vi "VisualizeCHROMA1.vi"() -> ()   [LabVIEW 2018, in "Visualization.lvlib" / "VisualizeAcPwr.lvclass"]
uses:
  VisualizeAcPwr.lvclass
  VisualizeBase/VisualizeBase_class/Requests/clUserEventType.ctl
  <vilib>/event_ctls.llb/usereventprio.ctl
  <vilib>/Utility/error.llb/Error Cluster From Error Code.vi
  <vilib>/ErrorRing/Error Ring.xnode
  VisualizeBase/VisualizeBase_class/VisualizeBase.lvclass
  <userlib>/NIST/NISTErrorLib/NISTErrorLib.lvlib
  AcPwr/AcPwrModule/AcPwrModule.lvlib
panel:
  in  "Tab Control":enum32{"Chart", "XY Graph"}(tab)
  out "Chroma":waveform(dbl)[](graph)=[{"t0"=timestamp(3659455182.3010225 s since 1904-01-01), "dt"=1.0, "Y"=[17.84]}, {"t0"=timestamp(3659455182.3010225 s since 1904-01-01), "dt"=1.0, "Y"=[3.99]}]
  in  "PlotYAxis":u32[](array[numeric])=[0, 1, 0] max=1
  out "Incorrect DataType?":bool
  out "Chroma's Internal Errors/Warnings":string="No Error"
  out "XY Graph":cluster{dbl[], dbl[]}(graph)={[0.02, 0.02, 0.02, 0.02, 0.02, 0.02, 0.02, 0.02, 0.1, 0.1, 0.1, 0.1, 0.1, 0.11, 0.2, 0.2, 0.2, 0.2, 0.2, 0.2, 0.3, 0.3, 0.3, 0.3, 0.3, 0.3, 0.3, 0.37, 0.4, 0.4, 0.4, 0.4, 0.4, 0.4, 0.48, 0.5, 0.5, 0.5, 0.5, 0.5, 0.5, 0.59, 0.6, 0.6, 0.6, 0.6, 0.6, 0.6, 0.6, 0.69, 0.69, 0.69, 0.69, 0.69, 0.69, 0.71, 0.79, 0.79, 0.79, 0.79, 0.79, 0.79, 0.89, 0.89, 0.89, 0.89, 0.89, 0.89, 0.89, 1.0, 1.0, 1.0, 1.0, 1.0, 1.0, 1.0, 1.1, 1.1, 1.1, 1.09, 1.09, 1.09, 1.1, 1.19, 1.19, 1.2, 1.2, 1.2, 1.2, 1.2, 1.29, 1.29, 1.29, 1.29, 1.29, 1.29, 1.29, 1.39, 1.39, 1.39, 1.39, 1.39, 1.39, 1.39, 1.4, 1.49, 1.49, 1.49, 1.49, 1.49, 1.49, 1.57, 1.59, 1.59, 1.59, 1.59, 1.59, 1.59, 1.69, 1.69, 1.69, 1.69, 1.69, 1.69, 1.69, 1.79, 1.79, 1.79, 1.79, 1.79, 1.79, 1.79, 1.89, 1.89, 1.89, 1.89, 1.89, 1.89, 1.89, 1.99, 1.99, 1.99, 1.99, 1.99, 1.99, 2.0, 2.09, 2.09, 2.09, 2.09, 2.09, 2.09, 2.13, 2.19, 2.19, 2.19, 2.19, 2.19, 2.19, 2.29, 2.29, 2.29, 2.29, 2.29, 2.29, 2.29, 2.29, 2.39, 2.39, 2.39, 2.39, 2.39, 2.39, 2.39, 2.49, 2.49, 2.49, 2.49, 2.49, 2.49, 2.51, 2.59, 2.59, 2.59, 2.59, 2.59, 2.59, 2.69, 2.69, 2.69, 2.69, 2.69, 2.69, 2.69, 2.79, 2.79, 2.79, 2.79, 2.79, 2.79, 2.79, 2.81, 2.89, 2.89, 2.89, 2.89, 2.89, 2.89, 2.89, 2.99, 2.99, 2.99, 2.99, 2.99, 2.99, 3.0, 3.09, 3.09, 3.09, 3.09, 3.09, 3.09, 3.1, 3.19, 3.19, 3.19, 3.19, 3.19, 3.19, 3.29, 3.29, 3.29, 3.29, 3.29, 3.29, 3.29, 3.39, 3.39, 3.39, 3.39, 3.39, 3.39, 3.39, 3.39, 3.49, 3.49, 3.49, 3.49, 3.49, 3.49, 3.49, 3.5, 3.59, 3.59, 3.59, 3.59, 3.59, 3.59, 3.6, 3.69, 3.69, 3.69, 3.69, 3.69, 3.69, 3.79, 3.79, 3.79, 3.79, 3.79, 3.79, 3.79, 3.89, 3.89, 3.89, 3.89, 3.89, 3.89, 3.89, 3.99, 3.99, 3.99, 3.99, 3.99, 3.99, 3.99], [42.02, 41.83, 42.15, 41.98, 41.52, 41.47, 41.64, 41.55, 41.51, 41.49, 41.46, 41.51, 41.41, 41.39, 41.42, 41.42, 41.41, 41.4, 41.29, 41.3, 41.32, 41.33, 41.32, 41.31, 41.32, 41.21, 41.21, 41.2, 41.2, 41.21, 41.22, 41.21, 41.1, 41.1, 41.09, 41.1, 41.09, 41.11, 41.1, 40.98, 40.99, 40.98, 40.98, 40.99, 40.99, 40.98, 40.98, 40.86, 40.86, 40.88, 40.87, 40.88, 40.87, 40.87, 40.74, 40.75, 40.75, 40.75, 40.73, 40.76, 40.63, 40.63, 40.62, 40.64, 40.64, 40.61, 40.64, 40.6, 40.5, 40.46, 40.5, 40.51, 40.5, 40.51, 40.37, 40.37, 40.37, 40.37, 40.37, 40.38, 40.37, 40.36, 40.22, 40.23, 40.23, 40.24, 40.23, 40.24, 40.1, 40.09, 40.07, 40.11, 40.09, 40.09, 40.11, 39.96, 39.96, 39.95, 39.96, 39.96, 39.96, 39.94, 39.81, 39.79, 39.79, 39.81, 39.8, 39.79, 39.79, 39.81, 39.65, 39.65, 39.65, 39.65, 39.64, 39.64, 39.65, 39.48, 39.48, 39.48, 39.48, 39.47, 39.48, 39.31, 39.31, 39.3, 39.31, 39.32, 39.31, 39.31, 39.14, 39.13, 39.13, 39.14, 39.13, 39.14, 39.13, 38.95, 38.95, 38.95, 38.94, 38.95, 38.95, 38.95, 38.75, 38.75, 38.76, 38.76, 38.75, 38.75, 38.75, 38.56, 38.56, 38.56, 38.56, 38.56, 38.55, 38.34, 38.34, 38.34, 38.33, 38.33, 38.34, 38.34, 38.11, 38.11, 38.1, 38.11, 38.12, 38.1, 38.11, 38.11, 37.87, 37.86, 37.86, 37.88, 37.86, 37.88, 37.86, 37.6, 37.61, 37.61, 37.61, 37.61, 37.61, 37.62, 37.33, 37.34, 37.33, 37.34, 37.34, 37.34, 37.04, 37.04, 37.05, 37.04, 37.06, 37.05, 37.04, 36.72, 36.72, 36.71, 36.72, 36.73, 36.72, 36.71, 36.72, 36.38, 36.37, 36.39, 36.37, 36.37, 36.38, 36.37, 36.0, 36.0, 35.99, 36.0, 35.99, 36.0, 35.99, 35.59, 35.59, 35.58, 35.58, 35.58, 35.58, 35.12, 35.12, 35.12, 35.13, 35.13, 35.13, 35.12, 34.6, 34.59, 34.59, 34.59, 34.59, 34.59, 34.59, 34.6, 33.97, 33.97, 33.98, 33.97, 33.98, 33.98, 33.98, 33.26, 33.27, 33.26, 33.26, 33.26, 33.26, 33.26, 33.26, 32.38, 32.39, 32.39, 32.37, 32.37, 32.39, 32.38, 31.25, 31.24, 31.25, 31.25, 31.25, 31.25, 29.64, 29.66, 29.66, 29.67, 29.65, 29.66, 29.66, 27.14, 27.15, 27.15, 27.15, 27.14, 27.14, 27.15, 17.86, 17.84]}
  in  "PluginName":string="AcPwr.Chroma1"
  out "ErrorArray":errorcluster[](array[cluster])
  in  "QueuName":string="CHROMADCVQ"
  in  "btnStop":bool
  in  "btnReset":bool
  in  "btnClear":bool
  # "0=Left Axis and 1=Right Axis"
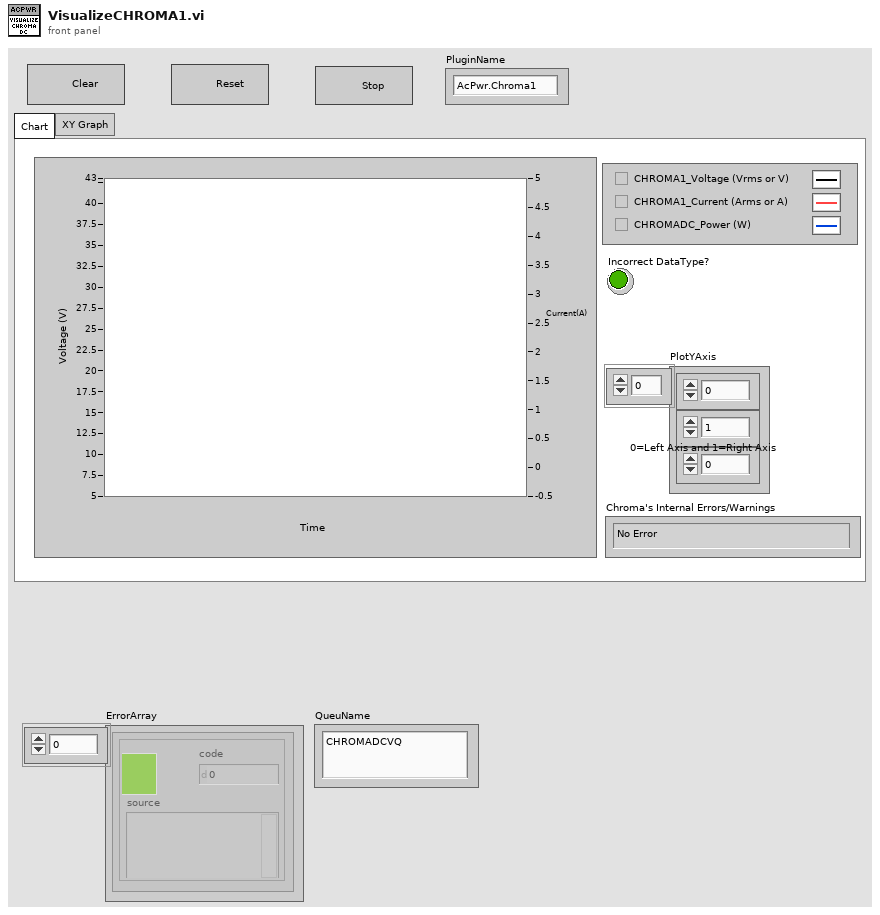
[diagram p1: front panel]
types:
  T1 = typedef "Visualization.lvlib/VisualizeBase.lvclass/clRequestEvents.ctl" = cluster{"StopRequest":refnum<user-event>, "ResetRequest":refnum<user-event>}
  T2 = typedef "AcPwrModule.lvlib/clBroadcastEvents.ctl" = cluster{"DidInit":refnum<user-event>, "StatusUpdate":refnum<user-event>, "ErrorReport":refnum<user-event>, "DidStop":refnum<user-event>, "PathToINI":refnum<user-event>, "Measurements":refnum<user-event>, "LoadConfigFile":refnum<user-event>, "GetSettings":refnum<user-event>, "SetSettings":refnum<user-event>, "GetType&ID":refnum<user-event>, "GotSettings":refnum<user-event>}
  T3 = typedef "Visualization.lvlib/VisualizeBase.lvclass/clUserEventType.ctl" = cluster{"BusIndex":i8, "Data":variant}
  T4 = typedef "usereventprio.ctl" = enum32{"high priority", "normal priority"}
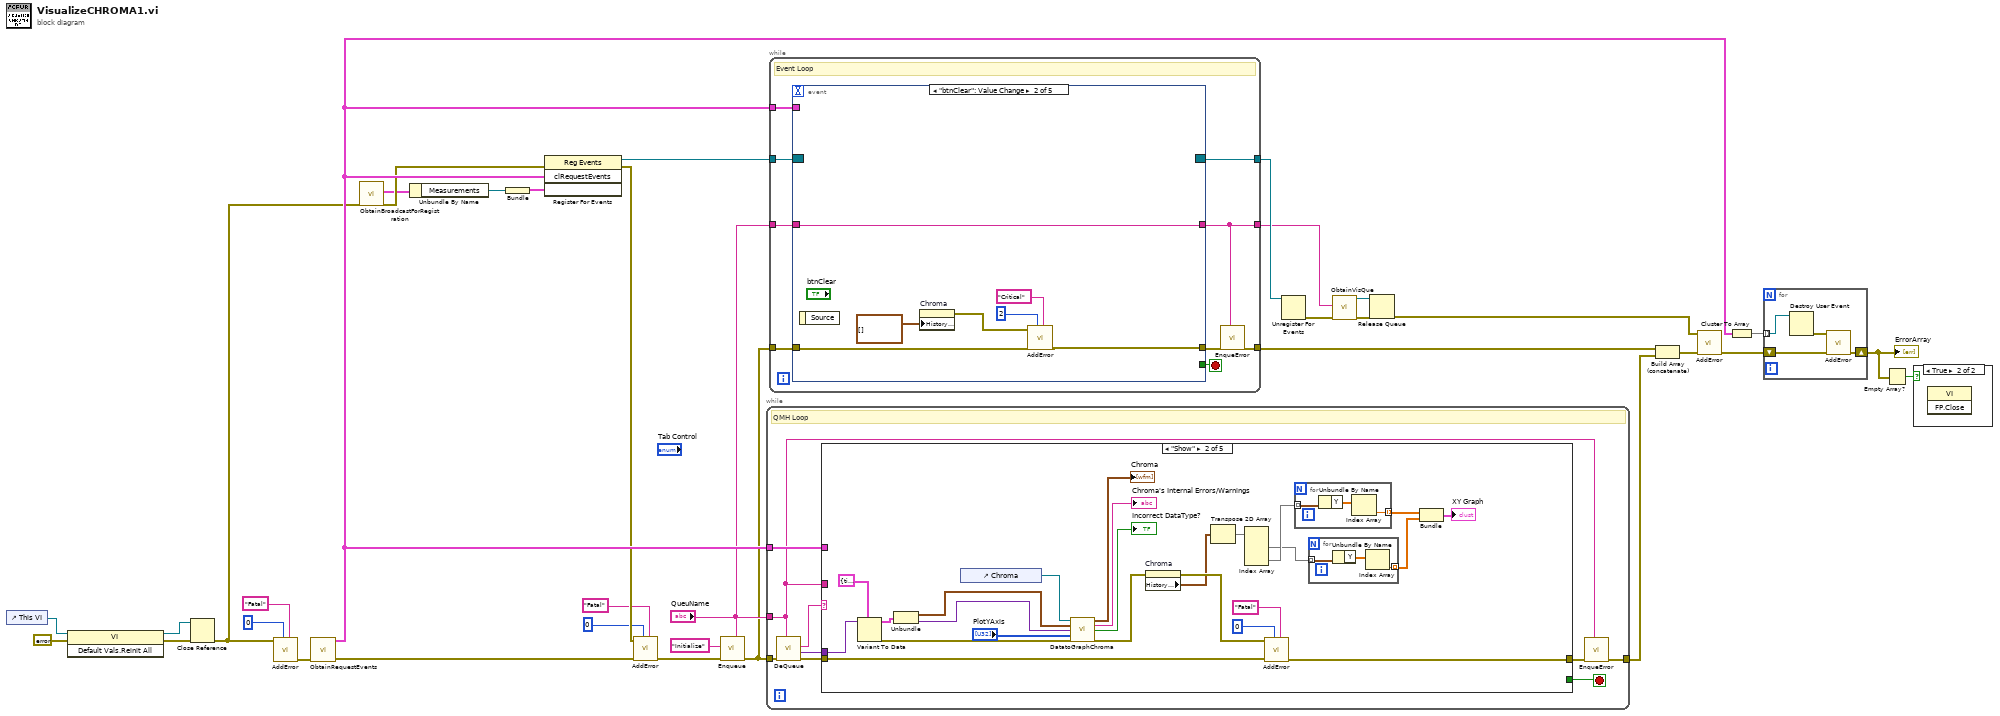
[diagram p0: block diagram]
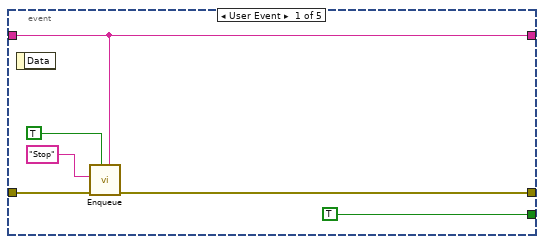
[diagram p2: hidden frame]
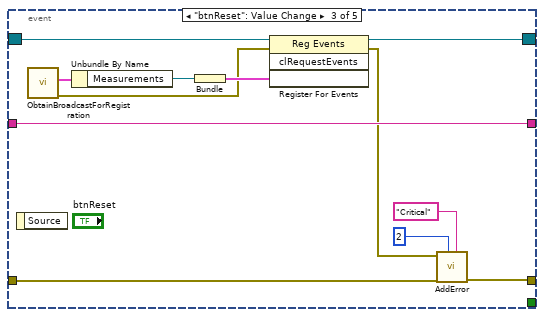
[diagram p3: hidden frame]
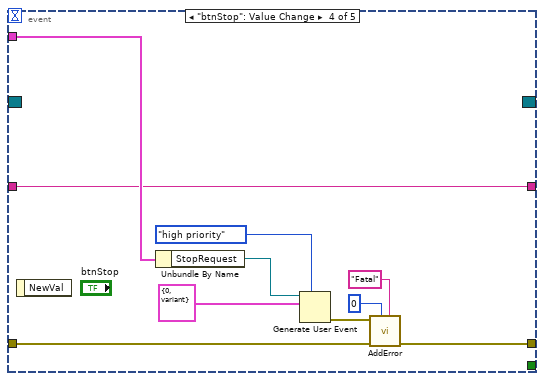
[diagram p4: hidden frame]
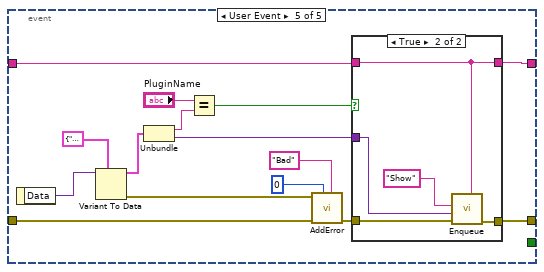
[diagram p5: hidden frame]
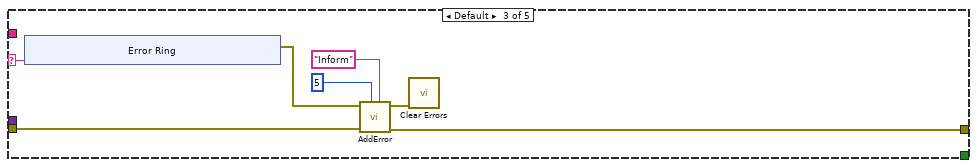
[diagram p9: hidden frame]
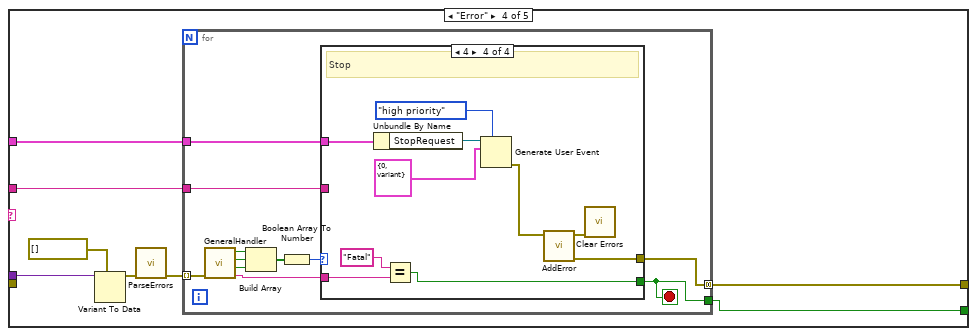
[diagram p10: hidden frame]
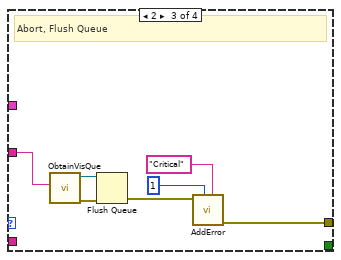
[diagram p13: hidden frame]
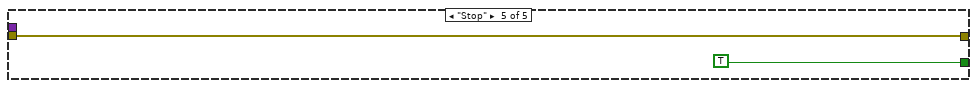
[diagram p14: hidden frame]
diagram:
  n1 = control-ref of="This VI"() -> (w18:refnum<vi>)
  n2 = invoke class="VI" method="Default Vals.Reinit All"(reference=w18, error in=errorcluster {"status"=FALSE, "code"=0, "source"=""} ("error in (no error)")) -> (reference out=w15:refnum<vi>, error out=w16:errorcluster)  [unwired: 1 in, 1 out]
  n3 = Close Reference(reference=w15, error in (no error)=w16) -> (error out=w13:errorcluster)
  n4 = call <userlib>:"AddError.vi"("Severity"="Fatal", "Priority"=u8 0, "error in (no error)"=w13) -> ("ErrorArray"=w33:errorcluster[])  [unwired: 7 in, 1 out]
  n5 = call "ObtainRequestEvents.vi"("Error"=w33) -> ("Error"=w7:errorcluster[], "clRequestEvents"=w22:T1)  [unwired: 9 in]
  n6 = call "ObtainBroadcastForRegistration.vi"("error in (no error)"=w13) -> ("error out"=w12:errorcluster, "clBroadcastEvents"=w11:T2)  [unwired: 9 in]
  n7 = Unbundle By Name(w11) -> ("Measurements"=w20:refnum<user-event>)
  n8 = Bundle("Measurements"=w20) -> (w19:cluster{"Measurements":refnum<user-event>})  [unwired: 1 in]
  n9 = register-events(error in=w12, w22, w19) -> (reference out=w34:refnum<event-registration>, error out=w4:errorcluster)  [unwired: 1 in]
  n10 = call <userlib>:"AddError.vi"("Severity"="Fatal", "Priority"=u8 0, "ErrorArray"=w7, "error in (no error)"=w4) -> ("ErrorArray"=w6:errorcluster[])  [unwired: 6 in, 1 out]
  n11 = call "Enqueue.vi"("QueName"="QueuName", "Error"=w6, "Message"="Initialize") -> ("Error"=w1:errorcluster[])  [unwired: 8 in]
  n12 = while {
    tunnel: w1 -> [w44]
    tunnel: [w38] -> w29
    tunnel: "QueuName" -> [w36]
    tunnel: w22 -> [w37]
    stop <- w39 stop-if-true
    # "QMH Loop"
    n13 = call "DeQueue.vi"("QueName"=w36, "Error"=w44) -> ("Error"=w41:errorcluster[], "Data"=w42:variant, "Message"=w43:string)  [unwired: 7 in]
    n14 = case shown="\"Show\"" w43 {
      selector: w43 -> [_ _ w82 _ _]
      tunnel: w42 -> [_ w66 _ w97 _]
      tunnel: w41 -> [w45 w63 w80 _ w126]
      tunnel: [w45 w69 w79 w93 w126] -> w40
      tunnel: [_ _ _ w92 TRUE] -> w39
      tunnel: w37 -> [_ _ _ w91 _]
      tunnel: w36 -> [_ _ _ w90 _]
      frame "Initialize" {
      }
      frame "Show" {
        n15 = Variant To Data(type=cluster{timestamp, "Data":variant} {timestamp(0 s since 1904-01-01), "Data"=variant}, Variant=w66) -> (data=w67:cluster{timestamp, "Data":variant}, error out=w65:errorcluster)  [unwired: 1 in]
        n16 = Unbundle(w67) -> (w57:timestamp, "Data"=w56:variant)
        n17 = control-ref of="Chroma"() -> (w68:refnum<vi>)
        n18 = call "DatatoGraphChroma.vi"("WaveformChartReference"=w68, "Time Stamp"=w57, "Data"=w56, "PlotYScale"="PlotYAxis", "error in (no error)"=w65) -> ("WaveformArray"=→"Chroma":waveform(dbl)[], "OutputString"=→"Chroma's Internal Errors/Warnings":string, "Incorrect DataType?"=→"Incorrect DataType?":bool, "error out"=w54:errorcluster)  [unwired: 7 in]
        n19 = property on="Chroma" class="WFChart (strict)"(error in=w54) -> (error out=w53:errorcluster, "History Data"=w52:waveform(dbl)[][])  [unwired: 1 in, 1 out]
        n20 = Transpose 2D Array(2D array=w52) -> (transposed array=w51:waveform(dbl)[][])
        n21 = Index Array(array=w51) -> (element #1=w48:waveform(dbl)[], element #2=w49:waveform(dbl)[])  [unwired: 4 in]
        n22 = call <userlib>:"AddError.vi"("Severity"="Fatal" ("String"), "Priority"=u8 0, "ErrorArray"=w63, "error in (no error)"=w53) -> ("ErrorArray"=w69:errorcluster[])  [unwired: 6 in, 1 out]
        n23 = for {
          tunnel: w49 -> [w75] mode=indexing
          tunnel: [w73] -> w46 mode=indexing
          n24 = Unbundle By Name(w75) -> ("Y"=w74:dbl[])
          n25 = Index Array(array=w74) -> (element=w73:dbl)  [unwired: 1 in]
        }
        n26 = for {
          tunnel: w48 -> [w72] mode=indexing
          tunnel: [w70] -> w47 mode=indexing
          n27 = Unbundle By Name(w72) -> ("Y"=w71:dbl[])
          n28 = Index Array(array=w71) -> (element=w70:dbl)  [unwired: 1 in]
        }
        n29 = Bundle(w46, w47) -> (→"XY Graph":cluster{dbl[], dbl[]})  [unwired: 1 in]
      }
      frame Default {
        n30 = xnode "Error Ring"("parameter 0"=w82) -> ("error out"=w81:errorcluster)
        n31 = call <userlib>:"AddError.vi"("Severity"="Inform" ("String"), "Priority"=u8 5, "ErrorArray"=w80, "error in (no error)"=w81) -> ("ErrorArray"=w79:errorcluster[], "error out"=w78:errorcluster)  [unwired: 6 in]
        n32 = call <vilib>:"Clear Errors.vi"("error in (no error)"=w78) -> ()  [unwired: 5 in, 2 out]
      }
      frame "Error" {
        n33 = Variant To Data(type=errorcluster[] [], Variant=w97) -> (data=w95:errorcluster[])  [unwired: 1 in, 1 out]
        n34 = call <userlib>:"ParseErrors.vi"("ErrorArray"=w95) -> ("ErrorArray"=w94:errorcluster[])  [unwired: 8 in, 2 out]
        n35 = for {
          tunnel: w94 -> [w108] mode=indexing
          tunnel: [w102] -> w93 mode=concatenating
          tunnel: [w100] -> w92
          tunnel: w91 -> [w99]
          tunnel: w90 -> [w98]
          stop <- w100 stop-if-true
          n36 = call <userlib>:"GeneralHandler.vi"("error in (no error)"=w108) -> ("Severity"=w101:string, "Stop"=w105:bool, "Abort"=w106:bool, "Continue"=w107:bool)  [unwired: 7 in]
          n37 = Build Array(w107, w106, w105) -> (w104:bool[])
          n38 = Boolean Array To Number(Boolean array=w104) -> (number=w103:u32)
          n39 = case shown="4" w103 {
            tunnel: [_ _ w113 w124] -> w102
            tunnel: w101 -> [_ _ _ w119]
            tunnel: [_ _ _ w117] -> w100
            tunnel: w99 -> [_ _ _ w116]
            tunnel: w98 -> [_ _ w109 _]
            frame 0, Default {
              # "No Dialog"
            }
            frame 1 {
              # "Continue"
            }
            frame 2 {
              # "Abort, Flush Queue"
              n40 = call "ObtainVisQue.vi"("QueName"=w109) -> ("error out"=w115:errorcluster, "queue out"=w114:refnum<queue>)  [unwired: 9 in]
              n41 = Flush Queue(queue=w114, error in (no error)=w115) -> (error out=w112:errorcluster)  [unwired: 2 out]
              n42 = call <userlib>:"AddError.vi"("Severity"="Critical" ("String"), "Priority"=u8 1, "error in (no error)"=w112) -> ("ErrorArray"=w113:errorcluster[])  [unwired: 7 in, 1 out]
            }
            frame 4 {
              # "Stop"
              n43 = Unbundle By Name(w116) -> ("StopRequest"=w125:refnum<user-event>)
              n44 = Equal?(x="Fatal", y=w119) -> (x = y?=w117:bool)
              n45 = Generate User Event(priority (normal)=usereventprio."high priority", user event=w125, event data cluster=T3 {"BusIndex"=0, "Data"=variant} ("event data")) -> (error out=w123:errorcluster)  [unwired: 1 in, 1 out]
              n46 = call <userlib>:"AddError.vi"("error in (no error)"=w123) -> ("ErrorArray"=w124:errorcluster[], "error out"=w120:errorcluster)  [unwired: 9 in]
              n47 = call <vilib>:"Clear Errors.vi"("error in (no error)"=w120) -> ()  [unwired: 5 in, 2 out]
            }
          }
        }
      }
      frame "Stop" {
      }
    }
    n48 = call "EnqueError.vi"("QueName"=w36, "Error"=w40) -> ("Error"=w38:errorcluster[])  [unwired: 9 in]
  }
  n49 = while {
    tunnel: w34 -> [w136]
    tunnel: [w133] -> w30
    tunnel: [w132] -> w32
    tunnel: w22 -> [w131]
    tunnel: w1 -> [w130]
    tunnel: "QueuName" -> [w129]
    tunnel: [w128] -> w9
    stop <- w135 stop-if-true
    # "Event Loop"
    n50 = event shown="[1] \"btnClear\": Value Change" {
      selector: w136 -> [_ _ w161 _ _]
      dyn-events: [_ _ w160 _ _] -> w132
      timeout: _ -> [_ _ _ _ _]
      tunnel: [TRUE _ _ _ _] -> w135
      tunnel: [w141 w145 w153 w169 w186] -> w134
      tunnel: w131 -> [_ _ _ w164 _]
      tunnel: w130 -> [w138 w146 w154 w162 w174]
      tunnel: w129 -> [w137 w149 w155 w163 w185]
      tunnel: [w137 w149 w155 w163 w177] -> w128
      event User Event {
        n51 = event-data() -> ()  [unwired: 1 in, 1 out]
        n52 = call "Enqueue.vi"("QueName"=w137, "Priority? (F)"=TRUE, "Error"=w138, "Message"="Stop") -> ("Error"=w141:errorcluster[])  [unwired: 7 in]
      }
      event "btnClear": Value Change {
        n53 = event-data() -> ()  [unwired: 1 in, 1 out]
        n54 = property on="Chroma" class="WFChart (strict)"("History Data"=waveform(dbl)[][] []) -> (error out=w144:errorcluster)  [unwired: 2 in, 1 out]
        n55 = call <userlib>:"AddError.vi"("Severity"="Critical", "Priority"=u8 2, "ErrorArray"=w146, "error in (no error)"=w144) -> ("ErrorArray"=w145:errorcluster[])  [unwired: 6 in, 1 out]
      }
      event "btnReset": Value Change {
        n56 = event-data() -> ()  [unwired: 1 in, 1 out]
        n57 = call "ObtainBroadcastForRegistration.vi"() -> ("error out"=w156:errorcluster, "clBroadcastEvents"=w157:T2)  [unwired: 10 in]
        n58 = Unbundle By Name(w157) -> ("Measurements"=w159:refnum<user-event>)
        n59 = Bundle("Measurements"=w159) -> (w158:cluster{"Measurements":refnum<user-event>})  [unwired: 1 in]
        n60 = register-events(reference=w161, error in=w156, w158) -> (reference out=w160:refnum<event-registration>, error out=w152:errorcluster)  [unwired: 1 in]
        n61 = call <userlib>:"AddError.vi"("Severity"="Critical", "Priority"=u8 2, "ErrorArray"=w154, "error in (no error)"=w152) -> ("ErrorArray"=w153:errorcluster[])  [unwired: 6 in, 1 out]
      }
      event "btnStop": Value Change {
        n62 = event-data() -> ()  [unwired: 1 in, 1 out]
        n63 = Unbundle By Name(w164) -> ("StopRequest"=w170:refnum<user-event>)
        n64 = Generate User Event(priority (normal)=usereventprio."high priority", user event=w170, event data cluster=T3 {"BusIndex"=0, "Data"=variant} ("event data")) -> (error out=w171:errorcluster)  [unwired: 1 in, 1 out]
        n65 = call <userlib>:"AddError.vi"("Severity"="Fatal" ("String"), "Priority"=u8 0, "ErrorArray"=w162, "error in (no error)"=w171) -> ("ErrorArray"=w169:errorcluster[])  [unwired: 6 in, 1 out]
      }
      event User Event {
        n66 = event-data() -> ("Data"=w183:variant)  [unwired: 1 in]
        n67 = Variant To Data(type=cluster{string, "Data":variant} {"", "Data"=variant}, Variant=w183) -> (data=w181:cluster{string, "Data":variant}, error out=w172:errorcluster)  [unwired: 1 in]
        n68 = Unbundle(w181) -> (w179:string, "Data"=w178:variant)
        n69 = Equal?(x="PluginName", y=w179) -> (x = y?=w184:bool)
        n70 = call <userlib>:"AddError.vi"("Severity"="Bad" ("String"), "Priority"=u8 0, "ErrorArray"=w174, "error in (no error)"=w172) -> ("ErrorArray"=w173:errorcluster[])  [unwired: 6 in, 1 out]
        n71 = case shown="True" w184 {
          tunnel: [w188 w192] -> w186
          tunnel: w185 -> [w187 w189]
          tunnel: w173 -> [w188 w191]
          tunnel: w178 -> [_ w190]
          tunnel: [w187 w189] -> w177
          frame False {
          }
          frame True {
            n72 = call "Enqueue.vi"("QueName"=w189, "Error"=w191, "Data"=w190, "Message"="Show") -> ("Error"=w192:errorcluster[])  [unwired: 7 in]
          }
        }
      }
    }
    n73 = call "EnqueError.vi"("QueName"=w128, "Error"=w134) -> ("Error"=w133:errorcluster[])  [unwired: 9 in]
  }
  n74 = Unregister For Events(event registration refnum=w32) -> (error out=w28:errorcluster)  [unwired: 1 in]
  n75 = call "ObtainVisQue.vi"("error in (no error)"=w28, "QueName"=w9) -> ("error out"=w26:errorcluster, "queue out"=w25:refnum<queue>)  [unwired: 8 in]
  n76 = Release Queue(queue=w25, error in (no error)=w26) -> (error out=w24:errorcluster)  [unwired: 1 in, 2 out]
  n77 = Build Array (concatenate)(w30, w29) -> (w27:errorcluster[])
  n78 = call <userlib>:"AddError.vi"("ErrorArray"=w27, "error in (no error)"=w24) -> ("ErrorArray"=w23:errorcluster[])  [unwired: 8 in, 1 out]
  n79 = Cluster To Array(cluster=w22) -> (array=w31:refnum<user-event>[])
  n80 = for {
    tunnel: w31 -> [w197] mode=indexing
    shift-right: [w196] -> w14
    shift-left: w23 -> [w195]
    n81 = Destroy User Event(user event=w197) -> (error out=w194:errorcluster)  [unwired: 1 in]
    n82 = call <userlib>:"AddError.vi"("ErrorArray"=w195, "error in (no error)"=w194) -> ("ErrorArray"=w196:errorcluster[])  [unwired: 8 in, 1 out]
  }
  "ErrorArray" <- w14
  n83 = Empty Array?(array=w14) -> (empty?=w21:bool)
  n84 = case shown="True" w21 {
    frame False {
    }
    frame True {
      n85 = invoke class="VI" method="FP.Close"() -> ()  [unwired: 3 in, 3 out]
    }
  }
